vi "VI Tree.vi"   [LabVIEW 2020, in "Keithley 27XX.lvlib"]
uses:
  <instrlib>/Keithley 27XX/Keithley 27XX.lvlib
  <instrlib>/Keithley 27XX/Public/Action-Status/Close Channel.vi
  <instrlib>/Keithley 27XX/Public/Configure/Measurement Specific/Configure Thermocouple.vi
  <instrlib>/Keithley 27XX/Public/Data/Read Multiple Direct.vi
panel:
  # "© 2005 National Instruments Corporation.  ALL RIGHTS RESERVED."
  # "VI TREE"
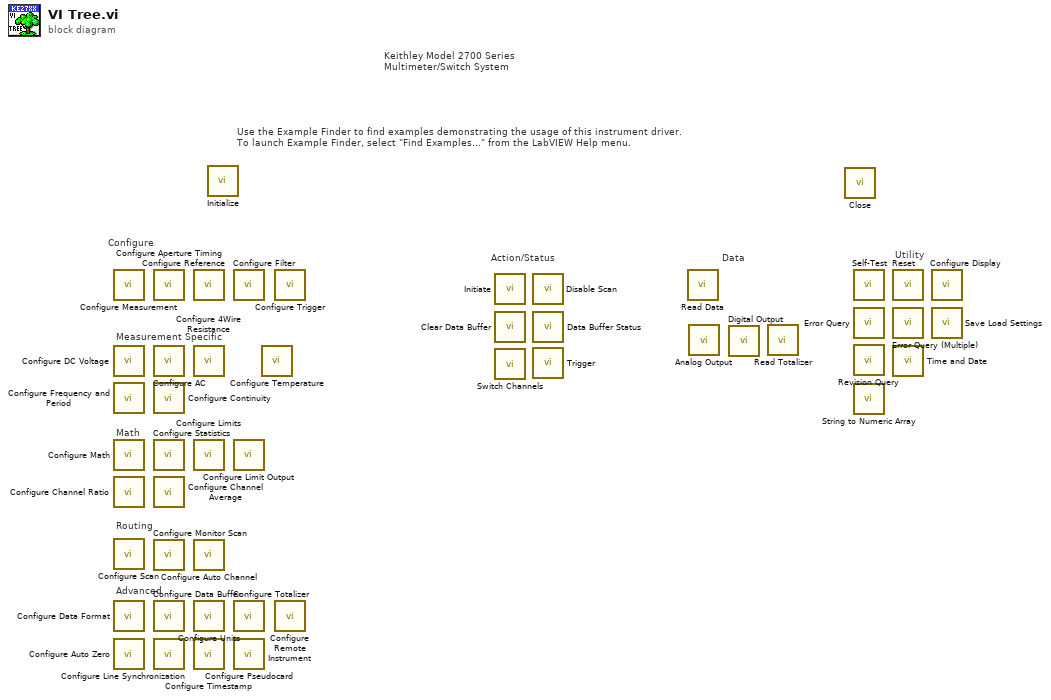
[diagram p0: block diagram]
diagram:
  # "Keithley Model 2700 Series\nMultimeter/Switch System"
  # "Configure"
  # "Advanced"
  # "Routing"
  # "Use the Example Finder to find examples demonstrating the usage of this instrument driver.\nTo launch Example Finder, select \"Find Examples...\" from the LabVIEW Help menu."
  # "Data"
  # "Math"
  # "Measurement Specific"
  # "Action/Status"
  # "Utility"
  n1 = call <instrlib>:"Configure Measurement.vi"() -> ()  [unwired: 14 in, 2 out]
  n2 = call <instrlib>:"Configure DC Voltage.vi"() -> ()  [unwired: 14 in, 2 out]
  n3 = call <instrlib>:"Configure Frequency and Period.vi"() -> ()  [unwired: 14 in, 2 out]
  n4 = call <instrlib>:"Configure Math.vi"() -> ()  [unwired: 18 in, 2 out]
  n5 = call <instrlib>:"Configure Channel Ratio.vi"() -> ()  [unwired: 14 in, 2 out]
  n6 = call <instrlib>:"Configure Scan.vi"() -> ()  [unwired: 14 in, 2 out]
  n7 = call <instrlib>:"Configure Data Format.vi"() -> ()  [unwired: 14 in, 2 out]
  n8 = call <instrlib>:"Configure Auto Zero.vi"() -> ()  [unwired: 14 in, 2 out]
  n9 = call <instrlib>:"Configure Aperture Timing.vi"() -> ()  [unwired: 14 in, 2 out]
  n10 = call <instrlib>:"Configure AC.vi"() -> ()  [unwired: 14 in, 2 out]
  n11 = call <instrlib>:"Configure Continuity.vi"() -> ()  [unwired: 14 in, 2 out]
  n12 = call <instrlib>:"Configure Statistics.vi"() -> ()  [unwired: 14 in, 2 out]
  n13 = call <instrlib>:"Configure Channel Average.vi"() -> ()  [unwired: 14 in, 2 out]
  n14 = call <instrlib>:"Configure Monitor Scan.vi"() -> ()  [unwired: 14 in, 2 out]
  n15 = call <instrlib>:"Configure Data Buffer.vi"() -> ()  [unwired: 14 in, 2 out]
  n16 = call <instrlib>:"Configure Line Synchronization.vi"() -> ()  [unwired: 14 in, 2 out]
  n17 = call <instrlib>:"Configure Reference.vi"() -> ()  [unwired: 14 in, 2 out]
  n18 = call <instrlib>:"Configure 4Wire Resistance.vi"() -> ()  [unwired: 14 in, 2 out]
  n19 = call <instrlib>:"Configure Limits.vi"() -> ()  [unwired: 18 in, 2 out]
  n20 = call <instrlib>:"Configure Auto Channel.vi"() -> ()  [unwired: 14 in, 2 out]
  n21 = call <instrlib>:"Configure Units.vi"() -> ()  [unwired: 14 in, 2 out]
  n22 = call <instrlib>:"Configure Timestamp.vi"() -> ()  [unwired: 14 in, 2 out]
  n23 = call <instrlib>:"Initialize.vi"() -> ()  [unwired: 14 in, 2 out]
  n24 = call <instrlib>:"Configure Filter.vi"() -> ()  [unwired: 14 in, 2 out]
  n25 = call <instrlib>:"Configure Limit Output.vi"() -> ()  [unwired: 14 in, 2 out]
  n26 = call <instrlib>:"Configure Totalizer.vi"() -> ()  [unwired: 14 in, 2 out]
  n27 = call <instrlib>:"Configure Pseudocard.vi"() -> ()  [unwired: 14 in, 2 out]
  n28 = call-poly <instrlib>:"Configure Temperature.vi"() -> ()  [unwired: 18 in, 2 out]
  n29 = call <instrlib>:"Configure Trigger.vi"() -> ()  [unwired: 14 in, 2 out]
  n30 = call <instrlib>:"Configure Remote Instrument.vi"() -> ()  [unwired: 14 in, 2 out]
  n31 = call <instrlib>:"Initiate.vi"() -> ()  [unwired: 14 in, 2 out]
  n32 = call <instrlib>:"Clear Data Buffer.vi"() -> ()  [unwired: 14 in, 2 out]
  n33 = call-poly <instrlib>:"Switch Channels.vi"() -> ()  [unwired: 14 in, 2 out]
  n34 = call <instrlib>:"Disable Scan.vi"() -> ()  [unwired: 14 in, 2 out]
  n35 = call <instrlib>:"Data Buffer Status.vi"() -> ()  [unwired: 11 in, 5 out]
  n36 = call <instrlib>:"Trigger.vi"() -> ()  [unwired: 14 in, 2 out]
  n37 = call-poly <instrlib>:"Read Data.vi"() -> ()  [unwired: 10 in, 6 out]
  n38 = call <instrlib>:"Analog Output.vi"() -> ()  [unwired: 14 in, 2 out]
  n39 = call <instrlib>:"Digital Output.vi"() -> ()  [unwired: 14 in, 2 out]
  n40 = call <instrlib>:"Read Totalizer.vi"() -> ()  [unwired: 13 in, 3 out]
  n41 = call <instrlib>:"Close.vi"() -> ()  [unwired: 15 in, 1 out]
  n42 = call <instrlib>:"Self-Test.vi"() -> ()  [unwired: 12 in, 4 out]
  n43 = call <instrlib>:"Error Query.vi"() -> ()  [unwired: 12 in, 4 out]
  n44 = call <instrlib>:"Revision Query.vi"() -> ()  [unwired: 8 in, 4 out]
  n45 = call <instrlib>:"String to Numeric Array.vi"() -> ()  [unwired: 11 in, 1 out]
  n46 = call <instrlib>:"Reset.vi"() -> ()  [unwired: 14 in, 2 out]
  n47 = call <instrlib>:"Error Query (Multiple).vi"() -> ()  [unwired: 12 in, 4 out]
  n48 = call <instrlib>:"Time and Date.vi"() -> ()  [unwired: 14 in, 2 out]
  n49 = call <instrlib>:"Configure Display.vi"() -> ()  [unwired: 14 in, 2 out]
  n50 = call <instrlib>:"Save Load Settings.vi"() -> ()  [unwired: 14 in, 2 out]
